vi "Channel Message Handler With Abort.vi"() -> ()   [LabVIEW 2023]
doc: "This template is for the Channel Message Handler design pattern.\n\nThe Event Handling Loop generates messages based on user interface actions.\n\nThe Message Handling Loop processes messages generated by the Event Handling Loop, or by other messages. The messages are string values, so new messages can be added easily to the Message Cases case structure in the Message Handling Loop. Each message cluster can also provide an optional value for Message Data, which is a variant that can be converted to whatever message-specific data is required."
uses:
  messages/MyMessage.lvclass/MyMessage.ctl
  messages/MyMessage.lvclass
  c:/dev/_r/4/eng/lv-core/lvpostprocessingd/lv_mc_x86_64/dist_i386/vi.lib/ChannelSupport/Channel Message/Channel Message.lvclass
  <vilib>/ChannelSupport/Channel Message/Channel Message.lvclass/Channel Message.ctl
  <vilib>/ChannelSupport/Channel Message/Read ID.vi
  <extravilib>/ChannelInstances/Stream-str/EndpointRead.vi
  <extravilib>/ChannelInstances/Stream-str/Endpoint.vi
  <extravilib>/ChannelInstances/Stream-str/Instantiate.vi
  <extravilib>/ChannelInstances/Stream-str/)Channel.vi
  <resource>/ChannelSupport/_ChannelSupport/WaitIfNeeded.vi
  <extravilib>/ChannelInstances/Messenger-class'MyMessage'/Instantiate.vi
  <extravilib>/ChannelInstances/Messenger-class'MyMessage'/Endpoint.vi
  <extravilib>/ChannelInstances/Stream-str.lvlib
  <extravilib>/ChannelInstances/Messenger-class'MyMessage'.lvlib
panel:
  in  "Exit flag":bool
  out "Status":string
  in  "Do Something Else <Replace Me>":bool
  in  "Do Something <Replace Me>":bool
  in  "Exit":bool
  # "These controls have associated \"Value Changed\" events configured in the Event Structure on the diagram.\n\nReplace them (and reconfigure the Event Structure) with the controls you need for your application."
  # "This template is for the Channel Message Handler design pattern.\n\nSee the block diagram for more information on how to use this template."
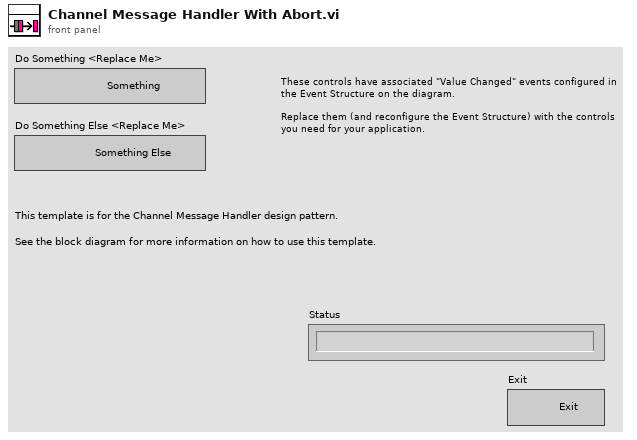
[diagram p1: front panel]
types:
  T1 = typedef "Messenger-class'MyMessage'.lvlib/))Channel.ctl" = refnum<queue>
  T2 = typedef "Stream-str.lvlib/)Channel.ctl" = refnum<queue>
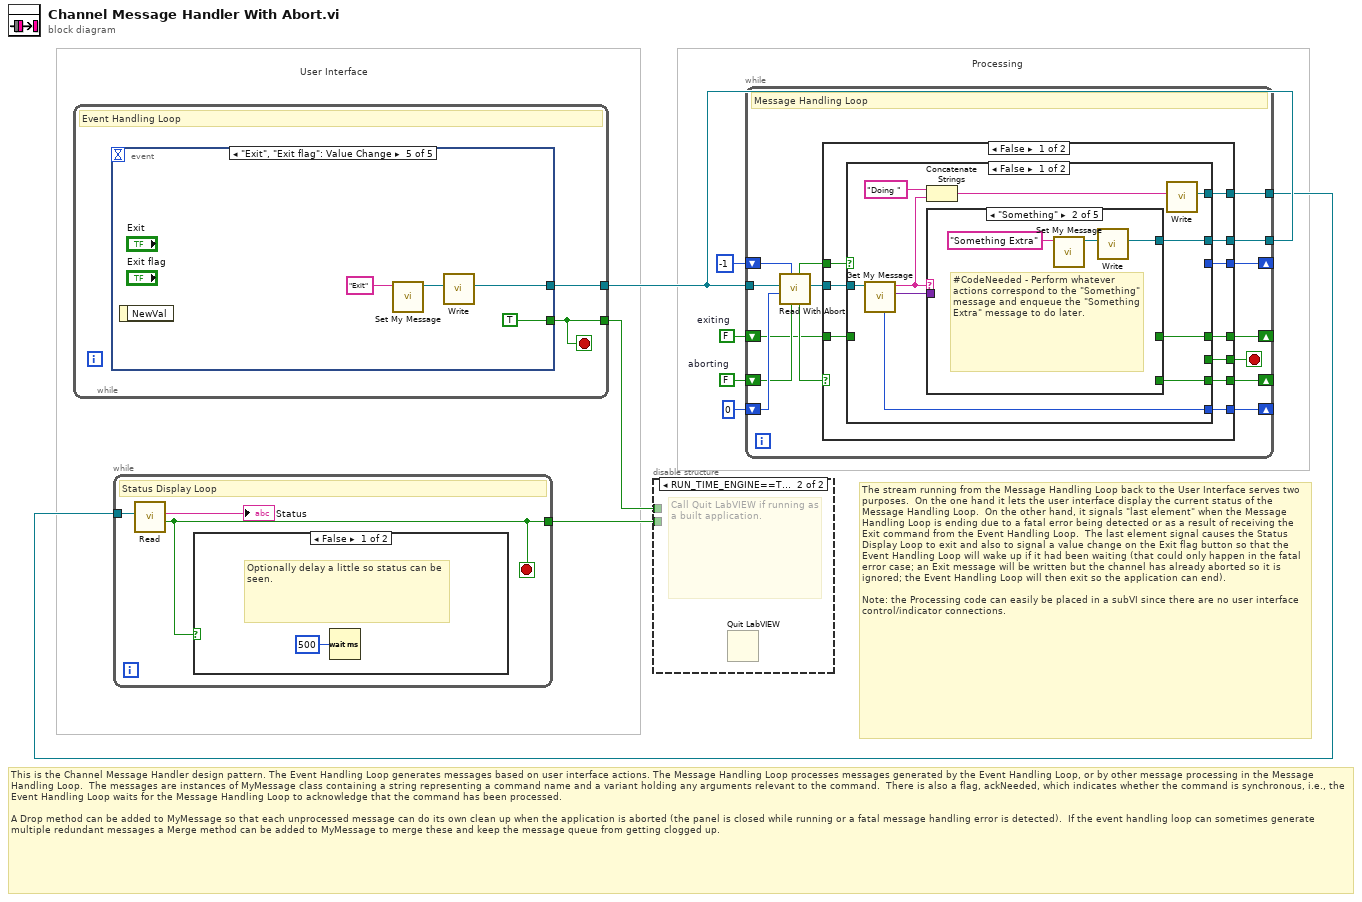
[diagram p0: block diagram]
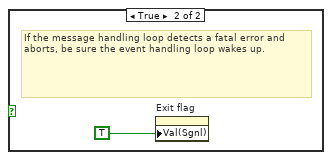
[diagram p2: hidden frame]
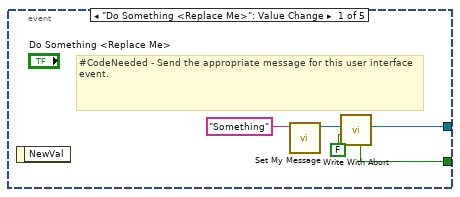
[diagram p4: hidden frame]
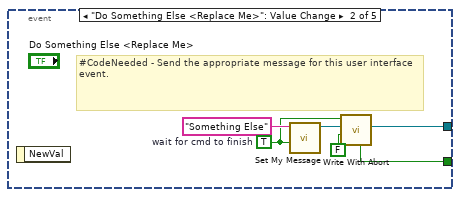
[diagram p5: hidden frame]
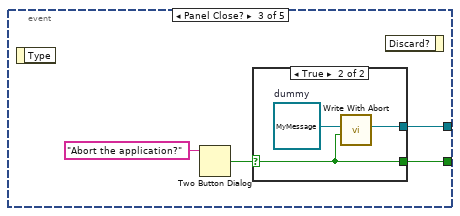
[diagram p6: hidden frame]
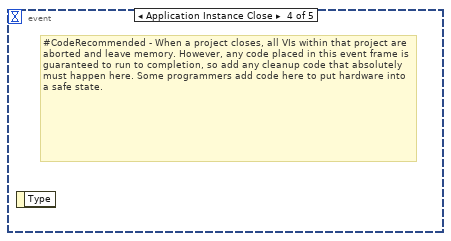
[diagram p8: hidden frame]
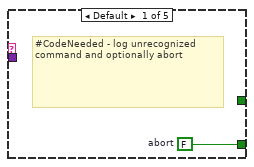
[diagram p9: hidden frame]
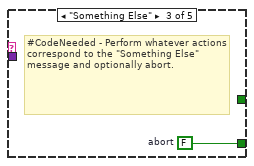
[diagram p10: hidden frame]
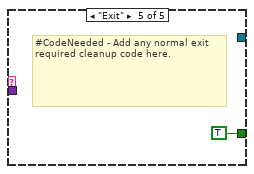
[diagram p12: hidden frame]
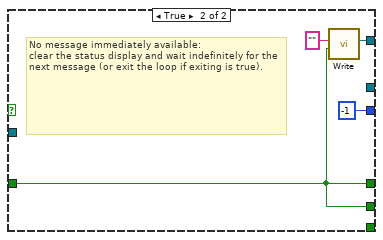
[diagram p13: hidden frame]
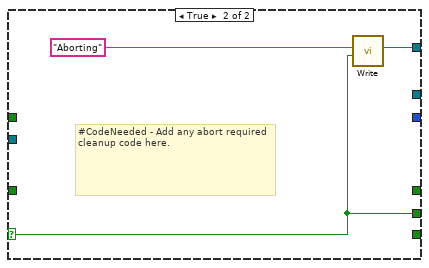
[diagram p14: hidden frame]
diagram:
  w1 = FALSE  # exiting
  w8 = FALSE  # aborting
  # "The stream running from the Message Handling Loop back to the User Interface serves two purposes.  On the one hand it lets the user interface display the current status of the Message Handling Loop.  On the other hand, it signals \"last element\" when the Message Handling Loop is ending due to a fatal error being detected or as a result of receiving the Exit command from the Event Handling Loop.  The last element signal causes the Status Display Loop to exit and also to signal a value change on the Exit flag button so that the Event Handling Loop will wake up if it had been waiting (that could only happen in the fatal error case; an Exit message will be written but the channel has already aborted so it is ignored; the Event Handling Loop will then exit so the application can end).\n\nNote: the Processing code can easily be placed in a subVI since there are no user interface control/indicator connections."
  # "Processing"
  # "User Interface"
  # "This is the Channel Message Handler design pattern. The Event Handling Loop generates messages based on user interface actions. The Message Handling Loop processes messages generated by the Event Handling Loop, or by other message processing in the Message Handling Loop.  The messages are instances of MyMessage class containing a string representing a command name and a variant holding any arguments relevant to the command.  There is also a flag, ackNeeded, which indicates whether the command is synchronous, i.e., the Event Handling Loop waits for the Message Handling Loop to acknowledge that the command has been processed.\n\nA Drop method can be added to MyMessage so that each unprocessed message can do its own clean up when the application is aborted (the panel is closed while running or a fatal message handling error is detected).  If the event handling loop can sometimes generate multiple redundant messages a Merge method can be added to MyMessage to merge these and keep the message queue from getting clogged up."
  n1 = while {
    tunnel: [w10] -> w6
    tunnel: [w9] -> w4
    stop <- w9 stop-if-true
    # "Event Handling Loop"
    n2 = event shown="[4] \"Exit\", \"Exit flag\": Value Change" {
      selector: _ -> [_ _ _ _ _]
      dyn-events: _ -> [_ _ _ _ _]
      timeout: _ -> [_ _ _ _ _]
      tunnel: [w12 w18 w22 _ TRUE] -> w9
      tunnel: [w13 w19 w24 _ w29] -> w10
      event "Do Something <Replace Me>": Value Change {
        # "#CodeNeeded - Send the appropriate message for this user interface event."
        n3 = event-data() -> ()  [unwired: 1 in, 1 out]
        n4 = call "Set My Message.vi"("command"="Something") -> ("MyMessage"=w14:refnum<class "MyMessage.lvclass">)  [unwired: 10 in]
        n5 = call <extravilib>:"Write With Abort.vi"("abort (F)"=FALSE, "element"=w14) -> ("channel"=w13:T1, "aborted?"=w12:bool)  [unwired: 6 in, 2 out]
      }
      event "Do Something Else <Replace Me>": Value Change {
        w17 = TRUE  # wait for cmd to finish
        # "#CodeNeeded - Send the appropriate message for this user interface event."
        n6 = event-data() -> ()  [unwired: 1 in, 1 out]
        n7 = call "Set My Message.vi"("ackNeeded"=w17, "command"="Something Else") -> ("MyMessage"=w20:refnum<class "MyMessage.lvclass">)  [unwired: 9 in]
        n8 = call <extravilib>:"Write With Abort.vi"("abort (F)"=FALSE, "element"=w20, "wait for ack (F)"=w17) -> ("channel"=w19:T1, "aborted?"=w18:bool)  [unwired: 5 in, 2 out]
      }
      event Panel Close? {
        n9 = event-data() -> ()  [unwired: 1 in, 1 out]
        n10 = Two Button Dialog(message="Abort the application?") -> (T button?=w23:bool)  [unwired: 2 in]
        n11 = case shown="True" w23 {
          selector: w23 -> [_ w26]
          tunnel: [_ w27] -> w24
          tunnel: [_ w26] -> w22
          frame False {
          }
          frame True {
            w28 = refnum<class "MyMessage.lvclass"> refnum  # dummy
            n12 = call <extravilib>:"Write With Abort.vi"("abort (F)"=w26, "element"=w28) -> ("channel"=w27:T1)  [unwired: 6 in, 3 out]
          }
        }
        n13 = event-data() -> ()  [unwired: 2 in, 1 out]
      }
      event Application Instance Close {
        # "#CodeRecommended - When a project closes, all VIs within that project are aborted and leave memory. However, any code placed in this event frame is guaranteed to run to completion, so add any cleanup code that absolutely must happen here. Some programmers add code here to put hardware into a safe state."
        n14 = event-data() -> ()  [unwired: 1 in, 1 out]
      }
      event "Exit", "Exit flag": Value Change {
        n15 = event-data() -> ()  [unwired: 1 in, 1 out]
        n16 = call "Set My Message.vi"("command"="Exit") -> ("MyMessage"=w30:refnum<class "MyMessage.lvclass">)  [unwired: 10 in]
        n17 = call <extravilib>:"Write.vi"("element"=w30) -> ("channel"=w29:T1)  [unwired: 8 in, 2 out]
      }
    }
  }
  n18 = while {
    tunnel: w6 -> [w47]
    shift-right: [w45] -> _
    shift-left: u32 0 ("id") -> [w44]
    shift-right: [w42] -> _
    shift-left: w8 -> [w41]
    tunnel: w6 -> [w40]
    tunnel: [w37] -> w5
    shift-right: [w35] -> _
    shift-left: -1 -> [w38]
    shift-right: [w34] -> _
    shift-left: w1 -> [w33]
    stop <- w39 stop-if-true
    # "Message Handling Loop"
    n19 = call <extravilib>:"Read With Abort.vi"("abort (F)"=w41, "timeout in ms (-1)"=w38, "ack id (0)"=w44, "channel"=w47) -> ("element"=w46:refnum<class "MyMessage.lvclass">, "aborted?"=w43:bool, "timed out?"=w36:bool)  [unwired: 4 in, 1 out]
    n20 = case shown="False" w43 {
      selector: w43 -> [_ w78]
      tunnel: w46 -> [w57 _]
      tunnel: [w56 _] -> w45
      tunnel: [w48 w78] -> w39
      tunnel: [w55 _] -> w42
      tunnel: [w54 _] -> w40
      tunnel: [w53 w80] -> w37
      tunnel: w36 -> [w52 _]
      tunnel: [w51 _] -> w35
      tunnel: [w50 _] -> w34
      tunnel: w33 -> [w49 _]
      frame False {
        n21 = case shown="False" w52 {
          tunnel: w57 -> [w67 _]
          tunnel: [w66 _] -> w56
          tunnel: [w64 _] -> w55
          tunnel: [w61 _] -> w54
          tunnel: [w59 w77] -> w53
          tunnel: [_ -1] -> w51
          tunnel: [w58 w74] -> w50
          tunnel: w49 -> [_ w74]
          tunnel: [_ w74] -> w48
          frame False {
            n22 = call "Get My Message.vi"("MyMessage"=w67) -> ("args"=w65:variant, "command"=w63:string, "id"=w66:u32)  [unwired: 7 in, 1 out]
            n23 = Concatenate Strings("Doing " ("string"), w63) -> (w60:string)
            n24 = case shown="\"Something\"" w63 {
              tunnel: w65 -> [_ _ _ _ _]
              tunnel: [_ _ _ _ TRUE] -> w58
              tunnel: [w68 _ w72 _ _] -> w64
              tunnel: [_ w69 _ _ _] -> w61
              frame Default {
                w68 = FALSE  # abort
                # "#CodeNeeded - log unrecognized command and optionally abort"
              }
              frame "Something" {
                # "#CodeNeeded - Perform whatever actions correspond to the \"Something\" message and enqueue the \"Something Extra\" message to do later."
                n25 = call "Set My Message.vi"("command"="Something Extra") -> ("MyMessage"=w71:refnum<class "MyMessage.lvclass">)  [unwired: 10 in]
                n26 = call <extravilib>:"Write.vi"("element"=w71) -> ("channel"=w69:T1)  [unwired: 8 in, 2 out]
              }
              frame "Something Else" {
                w72 = FALSE  # abort
                # "#CodeNeeded - Perform whatever actions correspond to the \"Something Else\" message and optionally abort."
              }
              frame "Something Extra" {
                # "#CodeNeeded - Perform whatever actions correspond to the \"Something Extra\" message."
              }
              frame "Exit" {
                # "#CodeNeeded - Add any normal exit required cleanup code here."
              }
            }
            n27 = call <extravilib>:"Write.vi"("element"=w60) -> ("channel"=w59:T2)  [unwired: 8 in, 2 out]
          }
          frame True {
            # "No message immediately available:\nclear the status display and wait indefinitely for the next message (or exit the loop if exiting is true)."
            n28 = call <extravilib>:"Write.vi"("last element? (F)"=w74, "element"="") -> ("channel"=w77:T2)  [unwired: 7 in, 2 out]
          }
        }
      }
      frame True {
        # "#CodeNeeded - Add any abort required cleanup code here."
        n29 = call <extravilib>:"Write.vi"("last element? (F)"=w78, "element"="Aborting") -> ("channel"=w80:T2)  [unwired: 7 in, 2 out]
      }
    }
  }
  n30 = while {
    tunnel: w5 -> [w83]
    tunnel: [w81] -> w3
    stop <- w81 stop-if-true
    # "Status Display Loop"
    n31 = call <extravilib>:"Read.vi"("channel"=w83) -> ("last element?"=w81:bool, "element"=→"Status":string)  [unwired: 6 in, 3 out]
    n32 = case shown="False" w81 {
      frame False {
        # "Optionally delay a little so status can be seen."
        n33 = Wait (ms)(milliseconds to wait=u32 500) -> ()  [unwired: 1 out]
      }
      frame True {
        # "If the message handling loop detects a fatal error and aborts, be sure the event handling loop wakes up."
        n34 = property on="Exit flag" class="Bool (strict)"("Val(Sgnl)"=TRUE) -> ()  [unwired: 2 in, 2 out]
      }
    }
  }
  n35 = disable-structure shown="RUN_TIME_ENGINE==True" {
    disable-tunnel: w4 -> [_ _]
    disable-tunnel: w3 -> [_ _]
    frame condition #0 (active) {
    }
    frame condition #1 {
      # "Call Quit LabVIEW if running as a built application."
      n36 = Quit LabVIEW() -> ()  [unwired: 1 in]
    }
  }
